vi "snake.add.vi"(8 "error in (no error)":errorcluster, 10 "Snake in":refnum<class "Snake.lvclass">, 11 "Game Board in":refnum<class "Game Board.lvclass">) -> (0 "error out":errorcluster, 3 "Game Board out":refnum<class "Game Board.lvclass">)   [LabVIEW 2020, in "Game Board.lvclass"]
uses:
  Game Board.lvclass
  Snake/Snake.lvclass
  Game Board.lvclass/Game Board.ctl
  Snake/Type Defs/Coordinates.ctl
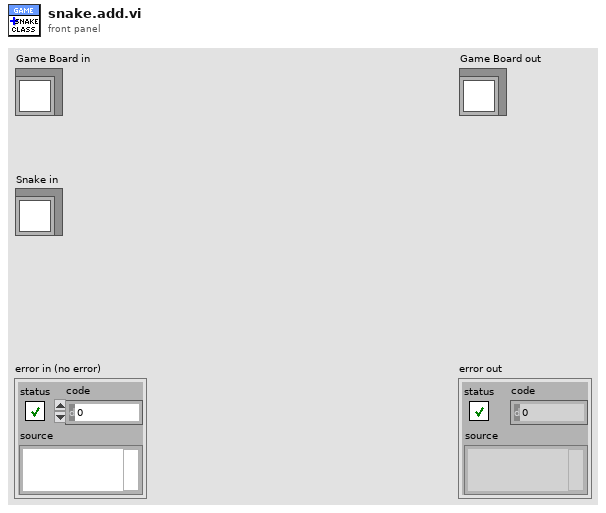
[diagram p1: front panel]
types:
  T1 = typedef "Coordinates.ctl" = cluster{"X":i32, "Y":i32}
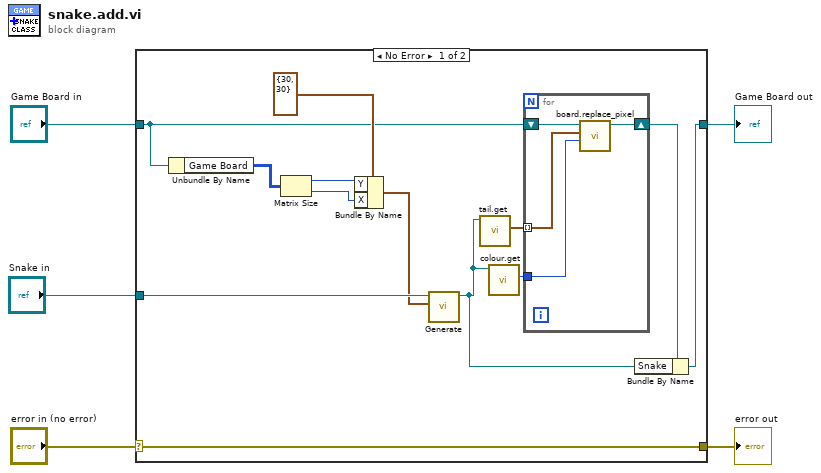
[diagram p0: block diagram]
diagram:
  n1 = case shown="No Error" "error in (no error)" {
    selector: "error in (no error)" -> [w18 w23]
    tunnel: [w18 w23] -> w4
    tunnel: [w7 w24] -> w2
    tunnel: "Game Board in" -> [w10 w24]
    tunnel: "Snake in" -> [w16 _]
    frame No Error {
      n2 = Unbundle By Name(w10) -> ("Game Board"=w17:u32[][])
      n3 = Matrix Size(0:w17) -> (1:w12:i32, 2:w13:i32)
      n4 = Bundle By Name(cluster=T1 {"X"=30, "Y"=30} ("Coordinates"), "Y"=w12, "X"=w13) -> (w14:T1)
      n5 = call "Generate.vi"("Coordinates"=w14, "Snake in"=w16) -> ("Snake out"=w6:refnum<class "Snake.lvclass">)  [unwired: 8 in, 1 out]
      n6 = call "tail.get.vi"("Snake in"=w6) -> ("Tail"=w11:T1[])  [unwired: 10 in]
      n7 = call-dynamic "colour.get.vi"("Game Componants in"=w6) -> ("Componant Colour"=w9:u32)  [unwired: 10 in]
      n8 = for {
        tunnel: w11 -> [w22] mode=indexing
        shift-right: [w20] -> w8
        shift-left: w10 -> [w21]
        tunnel: w9 -> [w19]
        n9 = call "board.replace_pixel.vi"("Colour"=w19, "Coordinates"=w22, "Game Board in"=w21) -> ("Game Board out"=w20:refnum<class "Game Board.lvclass">)  [unwired: 7 in, 1 out]
      }
      n10 = Bundle By Name(cluster=w8, "Snake"=w6) -> (w7:refnum<class "Game Board.lvclass">)
    }
    frame Error {
    }
  }
  "error out" <- w4
  "Game Board out" <- w2
